vi "Refresh_SubPanels.vi"(8 "error in (no error)":errorcluster, 9 "Root Container":refnum<vi>, 11 "Item_Refnums_Array":T1[](array[typedef])) -> (0 "error out":errorcluster, 3 "Item_Refnums_Array Out":T1[](array[typedef]))   [LabVIEW 2011, in "Root_XControl.xctl"]
uses:
  Root_XControl.xctl
  Controls/References/Item_Refnums.ctl
  Controls/References/Item_Command_Refnum.ctl
  Controls/Item_Command_Enum.ctl
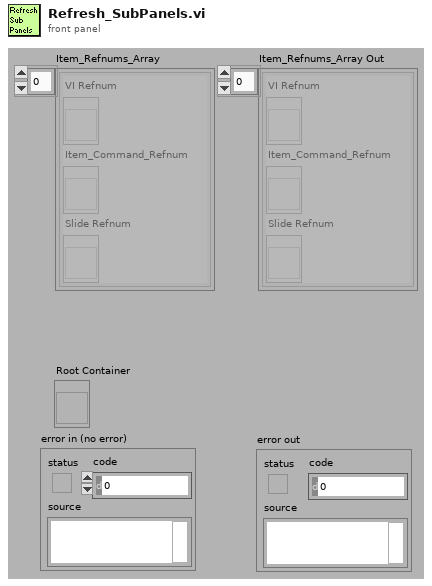
[diagram p1: front panel]
types:
  T1 = typedef "Item_Refnums.ctl" = cluster{"VI Refnum":refnum<vi>, "Item_Command_Refnum":T2, "Slide Refnum":refnum<vi>}
  T2 = typedef "Item_Command_Refnum.ctl" = refnum<vi>
  T3 = typedef "Item_Command_Enum.ctl" = enum16{"Stop", "Insert into Subpanel", "Update Value", "Remove from Subpanel"}
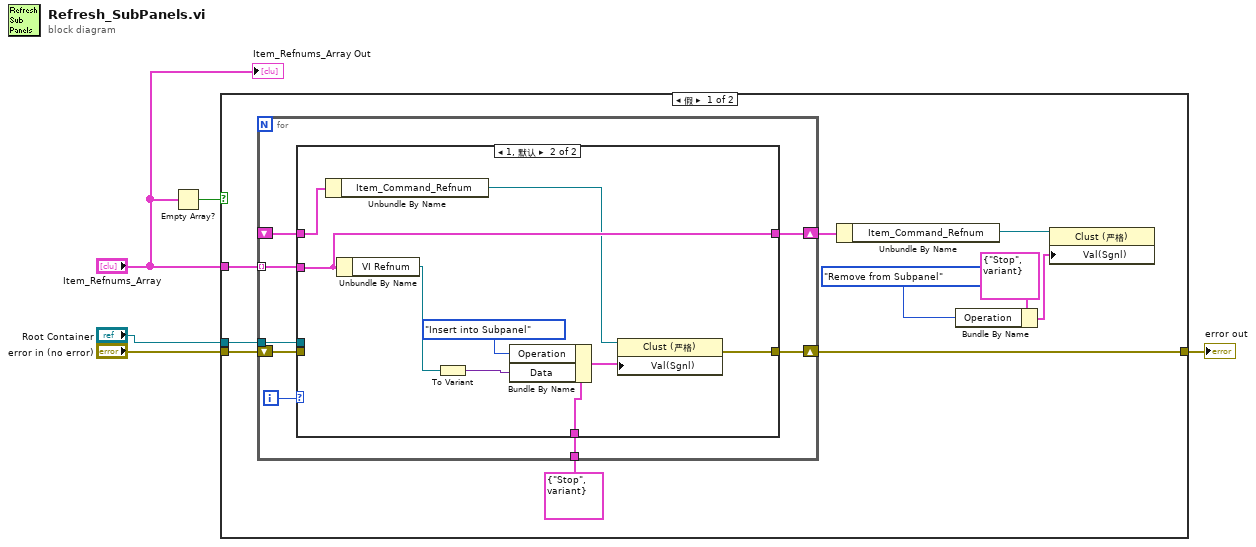
[diagram p0: block diagram]
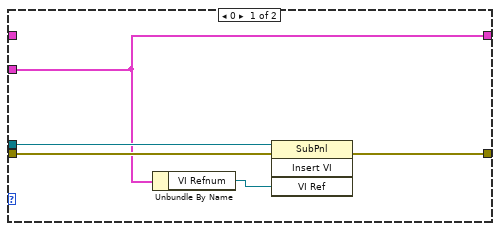
[diagram p2: hidden frame]
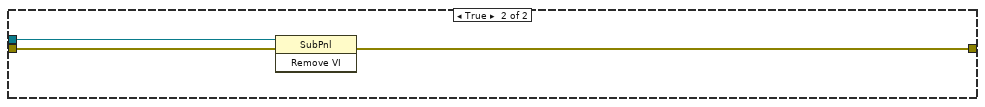
[diagram p3: hidden frame]
diagram:
  n1 = Empty Array?(array="Item_Refnums_Array") -> (empty?=w2:bool)
  n2 = case shown="假" w2 {
    tunnel: "Root Container" -> [w15 w40]
    tunnel: "Item_Refnums_Array" -> [w14 _]
    tunnel: "error in (no error)" -> [w12 w39]
    tunnel: [w11 w38] -> w3
    frame False {
      n3 = for {
        tunnel: w14 -> [w22] mode=indexing
        tunnel: w15 -> [w23]
        tunnel: cluster{"Operation":T3, "Data":variant} {"Operation"=enum."Stop", "Data"=variant} ("Item_Command") -> [w20]
        shift-right: [w18] -> w11
        shift-left: w12 -> [w19]
        shift-right: [w16] -> w6
        shift-left: _ -> [w17]
        i -> [w21]
        n4 = case shown="1, 默认" w21 {
          tunnel: w22 -> [w24 w37]
          tunnel: w23 -> [w28 _]
          tunnel: w20 -> [_ w33]
          tunnel: w19 -> [w27 _]
          tunnel: [w26 w32] -> w18
          tunnel: w17 -> [_ w31]
          tunnel: [w24 w37] -> w16
          frame 0 {
            n5 = Unbundle By Name(w24) -> ("VI Refnum"=w25:refnum<vi>)
            n6 = invoke on="Invoke Node" class="SubPnl" method="Insert VI"(reference=w28, error in=w27, "VI Ref"=w25) -> (error out=w26:errorcluster)  [unwired: 1 in, 3 out]
          }
          frame 1, Default {
            n7 = Unbundle By Name(w31) -> ("Item_Command_Refnum"=w35:T2)
            n8 = Unbundle By Name(w37) -> ("VI Refnum"=w30:refnum<vi>)
            n9 = To Variant(anything=w30) -> (Variant=w29:variant)
            n10 = Bundle By Name(cluster=w33, "Operation"=Item_Command_Enum."Insert into Subpanel", "Data"=w29) -> (w34:cluster{"Operation":T3, "Data":variant})
            n11 = property class="Clust (严格)"(reference=w35, "Val(Sgnl)"=w34) -> (error out=w32:errorcluster)  [unwired: 1 in, 1 out]
          }
        }
      }
      n12 = Unbundle By Name(w6) -> ("Item_Command_Refnum"=w10:T2)
      n13 = Bundle By Name(cluster=cluster{"Operation":T3, "Data":variant} {"Operation"=enum."Stop", "Data"=variant} ("Item_Command"), "Operation"=Item_Command_Enum."Remove from Subpanel") -> (w8:cluster{"Operation":T3, "Data":variant})
      n14 = property class="Clust (严格)"(reference=w10, "Val(Sgnl)"=w8) -> ()  [unwired: 1 in, 2 out]
    }
    frame True {
      n15 = invoke on="Invoke Node" class="SubPnl" method="Remove VI"(reference=w40, error in=w39) -> (error out=w38:errorcluster)  [unwired: 1 in, 2 out]
    }
  }
  "error out" <- w3
  "Item_Refnums_Array Out" <- "Item_Refnums_Array"
